vi "PI POS.vi"(8 "error in (no error)":errorcluster, 10 "query":string="POS? A", 11 "ID in":i32) -> (0 "error out":errorcluster, 2 "Position":dbl, 3 "ID out":i32)   [LabVIEW 2020]
uses:
  Low Level/GCSTranslator.dll
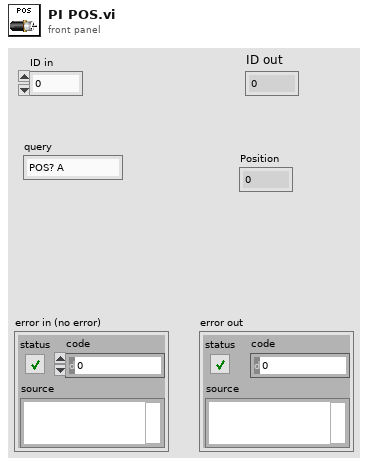
[diagram p1: front panel]
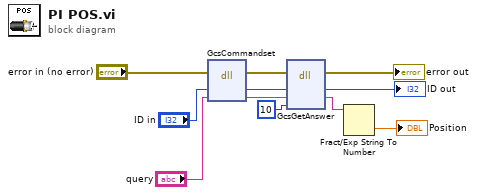
[diagram p0: block diagram]
diagram:
  n1 = dll-call lib="D:/software/TweezerTron Project/Instruments/Physik Instrumente/SDK/GCS_LabVIEW_digital/Low Level/GCSTranslator.dll" fn="GcsCommandset" ("POS")(error in="error in (no error)", "ID"="ID in", "szCommand"="query") -> (error out=w4:errorcluster, "ID"=w9:i32, "szCommand"=w8:string)  [unwired: 2 in, 2 out]
  n2 = dll-call lib="D:/software/TweezerTron Project/Instruments/Physik Instrumente/SDK/GCS_LabVIEW_digital/Low Level/GCSTranslator.dll" fn="GcsGetAnswer"(error in=w4, "ID"=w9, "szAnswer"=w8, "iAnswerSize"=10) -> (error out=→"error out":errorcluster, "ID"=→"ID out":i32, "szAnswer"=w3:string)  [unwired: 3 in, 2 out]
  n3 = Fract/Exp String To Number(string=w3) -> (number=→"Position":dbl)  [unwired: 3 in, 1 out]
